vi "缺陷评定结果显示子VI.vi"(6 "疑似分层类缺陷数":dbl, 7 "不合格缺陷数":dbl, 8 "疏松类缺陷数":dbl, 9 "其它缺陷数":dbl, 10 "总缺陷数":dbl, 11 "评定结果":dbl[][](array[numeric])) -> (3 "缺陷最终评定结果":T1)   [LabVIEW 2018]
panel:
  out "不合格缺陷个数":dbl
  out "其它不明显缺陷个数":dbl
  out "疑似分层类缺陷个数":dbl
  out "疏松类缺陷个数":dbl
  out "总缺陷个数":dbl
  in  "退出":bool
  out "评定结果显示表":dbl[][](array[numeric])
  # "缺陷评定结果显示表"
  # "缺陷编号"
  # "缺陷位置_X"
  # "缺陷位置_Y"
  # "缺陷长度(mm)"
  # "缺陷宽度(mm)"
  # "最大灰度值"
  # "最小灰度值"
  # "缺陷面积（mm2）"
  # "缺陷Z值（mm）"
  # "缺陷部位"
  # "缺陷性质"
  # "缺陷合格性"
  # "备注：\n（1）缺陷部位：0—蒙皮部位、1—筋条部位；\n（2）缺陷性质：1—疏松类缺陷、2—疑似分层类缺陷、0—其它轻微缺陷；\n（3）缺陷合格性：1—不合格、0—合格。"
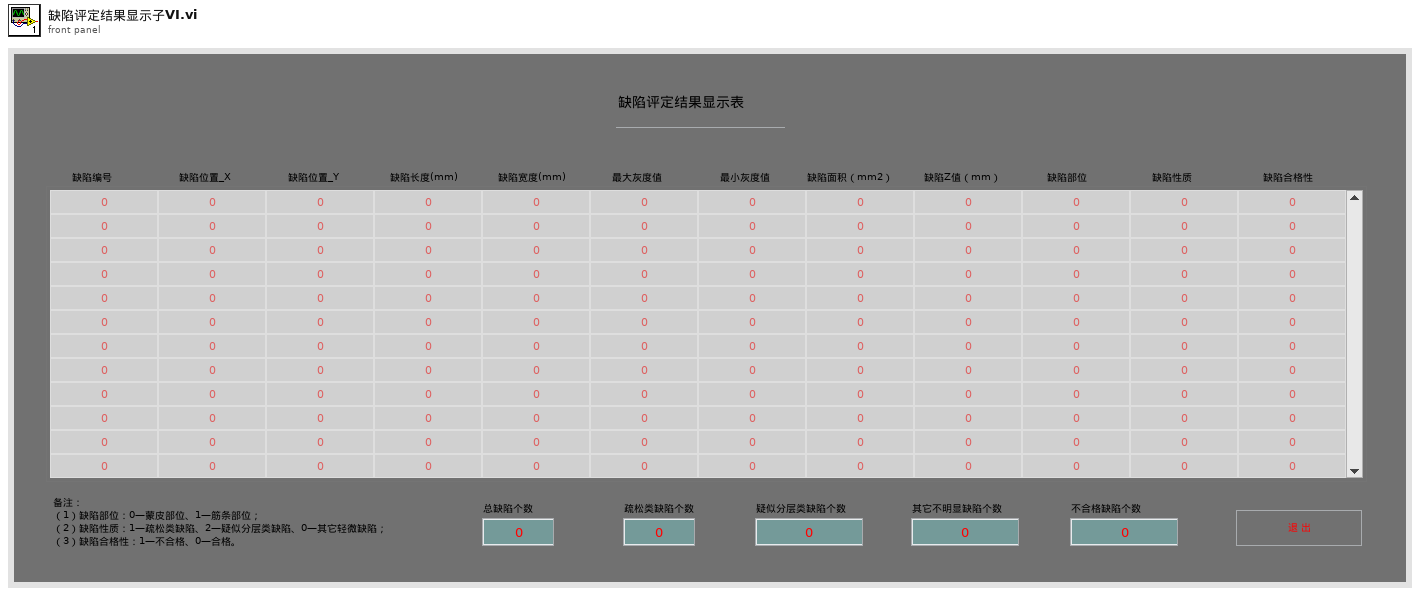
[diagram p1: front panel]
types:
  T1 = cluster{"总缺陷数":dbl, "疏松类缺陷数":dbl, "疑似分层类缺陷数":dbl, "其它缺陷数":dbl, "不合格缺陷数":dbl, "评定结果":dbl[][]}
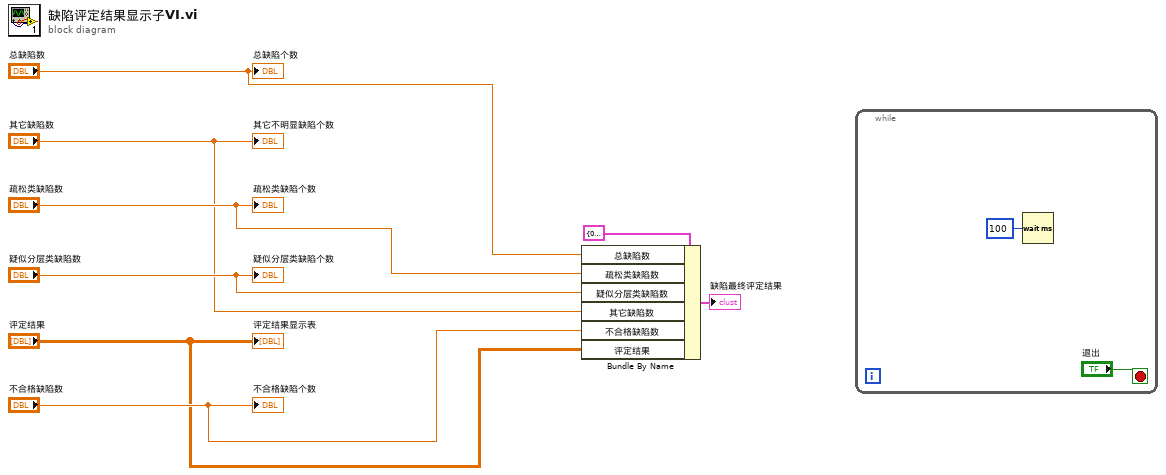
[diagram p0: block diagram]
diagram:
  n1 = Bundle By Name(cluster=T1 {"总缺陷数"=0.0, "疏松类缺陷数"=0.0, "疑似分层类缺陷数"=0.0, "其它缺陷数"=0.0, "不合格缺陷数"=0.0, "评定结果"=[]} ("簇"), "总缺陷数"="总缺陷数", "疏松类缺陷数"="疏松类缺陷数", "疑似分层类缺陷数"="疑似分层类缺陷数", "其它缺陷数"="其它缺陷数", "不合格缺陷数"="不合格缺陷数", "评定结果"="评定结果") -> (→"缺陷最终评定结果":T1)
  n2 = while {
    stop <- "退出" stop-if-true
    n3 = Wait (ms)(milliseconds to wait=u32 100 ("等待时间（毫秒）")) -> ()  [unwired: 1 out]
  }
  "评定结果显示表" <- "评定结果"
  "其它不明显缺陷个数" <- "其它缺陷数"
  "疑似分层类缺陷个数" <- "疑似分层类缺陷数"
  "总缺陷个数" <- "总缺陷数"
  "疏松类缺陷个数" <- "疏松类缺陷数"
  "不合格缺陷个数" <- "不合格缺陷数"
